vi "fgv_DL950_data.vi"(7 "cmd":T2, 8 "error in":errorcluster, 11 "DL950 wfm":T1={"wfms"=[], "Waveform_2"={"t0"=0.0, "dt"=0.0, "Y"=[]}, "items"=[], "da950_array"=[10.0, 0.02, 0.074492, 0.033331, 0.018948904, 3.5928321, 0.0, 0.0, 400.375, 399.625, 3.5928321, 0.0, 0.0, 0.074492, 0.0, 0.0]}) -> (0 "error out":errorcluster, 3 "DL950 wfm 2":T1={"wfms"=[], "Waveform_2"={"t0"=0.0, "dt"=0.0, "Y"=[]}, "items"=[], "da950_array"=[10.0, 0.02, 0.074492, 0.033331, 0.018948904, 3.5928321, 0.0, 0.0, 400.375, 399.625, 3.5928321, 0.0, 0.0, 0.074492, 0.0, 0.0]})   [LabVIEW 2019]
uses:
  _ctrl/rw.ctl
  Durability/DL950_wfms.ctl
panel:
  out "wfm1":waveform(dbl)[](array[waveform])
  out "wfms 2":waveform(dbl)[](array[waveform])
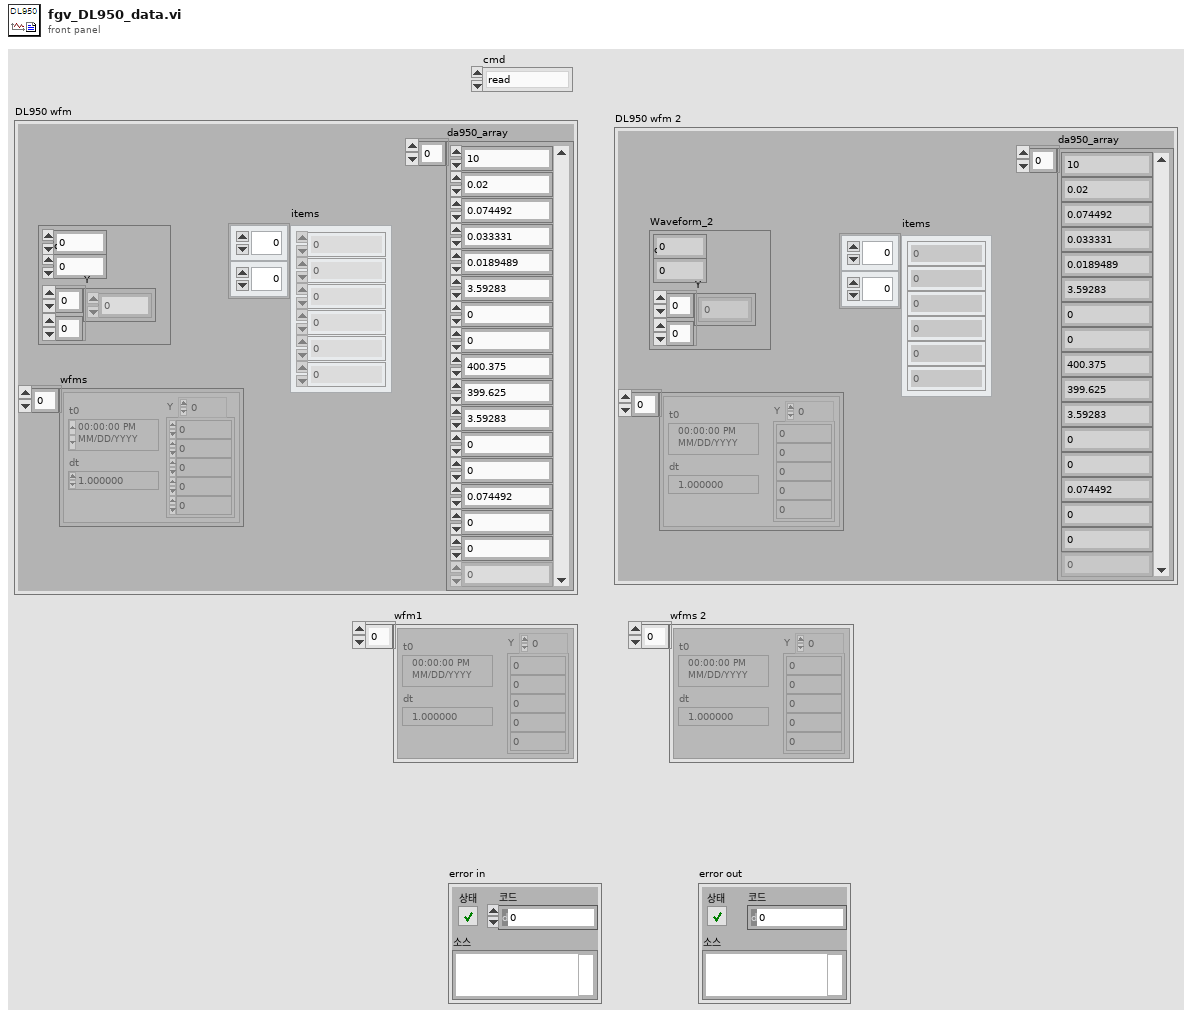
[diagram p1: front panel]
types:
  T1 = typedef "DL950_wfms.ctl" = cluster{"wfms":waveform(dbl)[], "Waveform_2":cluster{"t0":dbl, "dt":dbl, "Y":dbl[][]}, "items":dbl[][], "da950_array":dbl[]}
  T2 = typedef "rw.ctl" = enum16{"read", "write"}
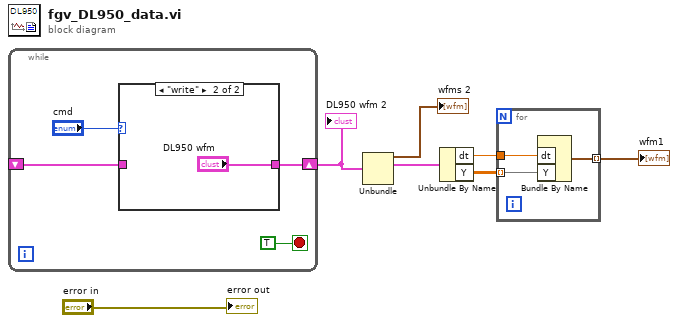
[diagram p0: block diagram]
diagram:
  n1 = while {
    shift-right: [w9] -> w3
    shift-left: _ -> [w8]
    stop <- TRUE stop-if-true
    n2 = case shown="\"write\"" "cmd" {
      tunnel: [w12 "DL950 wfm"] -> w9
      tunnel: w8 -> [w12 _]
      frame "read", Default {
      }
      frame "write" {
      }
    }
  }
  "DL950 wfm 2" <- w3
  n3 = Unbundle(w3) -> ("wfms"=→"wfms 2":waveform(dbl)[], "Waveform_2"=w1:cluster{"t0":dbl, "dt":dbl, "Y":dbl[][]})  [unwired: 2 out]
  n4 = Unbundle By Name(w1) -> ("dt"=w5:dbl, "Y"=w6:dbl[][])
  n5 = for {
    tunnel: w6 -> [w15] mode=indexing
    tunnel: w5 -> [w16]
    tunnel: [w14] -> w4 mode=indexing
    n6 = Bundle By Name("dt"=w16, "Y"=w15) -> (w14:waveform(dbl))  [unwired: 1 in]
  }
  "wfm1" <- w4
  "error out" <- "error in"
